vi "Get visa 1d DBL data.vi"(7 "VISA resource name":refnum<visa-resource-name>, 8 "error in (no error)":errorcluster, 9 "Name":string, 10 "Mag Lab Parameters in":refnum<class "Mag Lab Parameters.lvclass">, 11 "Oxford Mercury IPS in":refnum<class "Oxford Mercury IPS.lvclass">) -> (0 "error out":errorcluster, 1 "Channel data":dbl[](array[numeric]), 2 "Channel names":string[](array[string]), 3 "Oxford Mercury IPS out":refnum<class "Oxford Mercury IPS.lvclass">, 5 "VISA resource name out":refnum<visa-resource-name>)   [LabVIEW 2015, in "Oxford Mercury IPS.lvclass"]
uses:
  Oxford Mercury IPS.lvclass
  Mag Lab Properties/Mag Lab Parameters.lvclass
  Instruments/GPIB/VISA  Send Receive.vi
panel:
  out "after substring":string
  out "data string out":string
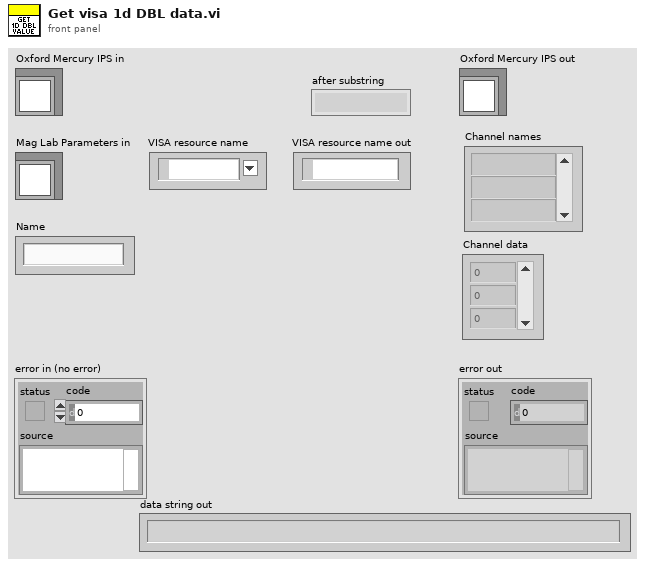
[diagram p1: front panel]
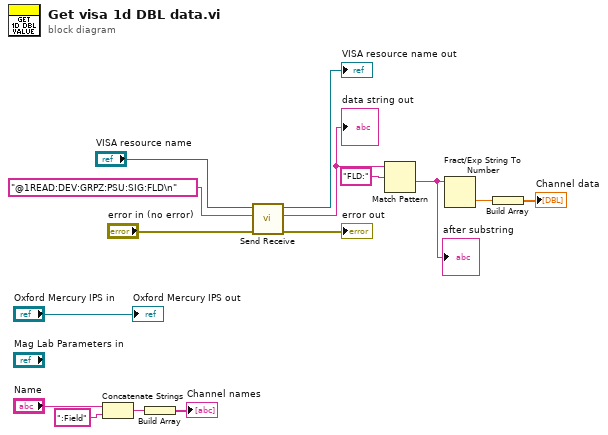
[diagram p0: block diagram]
diagram:
  n1 = Concatenate Strings("Name", ":Field" ("string")) -> (w13:string)
  n2 = Build Array(w13) -> (→"Channel names":string[])
  n3 = call-poly "Send Receive.vi"("error in (no error)"="error in (no error)", "data string in"="@1READ:DEV:GRPZ:PSU:SIG:FLD\n", "VISA Resource Name"="VISA resource name") -> ("error out"=→"error out":errorcluster, "data string out"=w5:string, "VISA Resource Name Out"=→"VISA resource name out":refnum<visa-resource-name>)  [unwired: 6 in]
  "data string out" <- w5
  n4 = Match Pattern(string=w5, regular expression="FLD:") -> (after substring=w3:string)  [unwired: 1 in, 3 out]
  "after substring" <- w3
  n5 = Fract/Exp String To Number(string=w3) -> (number=w2:dbl)  [unwired: 3 in, 1 out]
  n6 = Build Array(w2) -> (→"Channel data":dbl[])
  "Oxford Mercury IPS out" <- "Oxford Mercury IPS in"
